vi "OTP - Verify data written.vi"(4 "Read Return":string[](array[string]), 6 "Write Return":string[](array[string]), 9 "Read in":T1[](array[typedef]), 11 "write in":T1[](array[typedef])) -> (0 "# of regs still to be written":i32, 1 "Read out":T1[](array[typedef]), 3 "write out":T1[](array[typedef]))   [LabVIEW 2020]
uses:
  Devices/Controls/Register to Write.ctl
  Devices/PIC-device/PIC-Device.lvclass
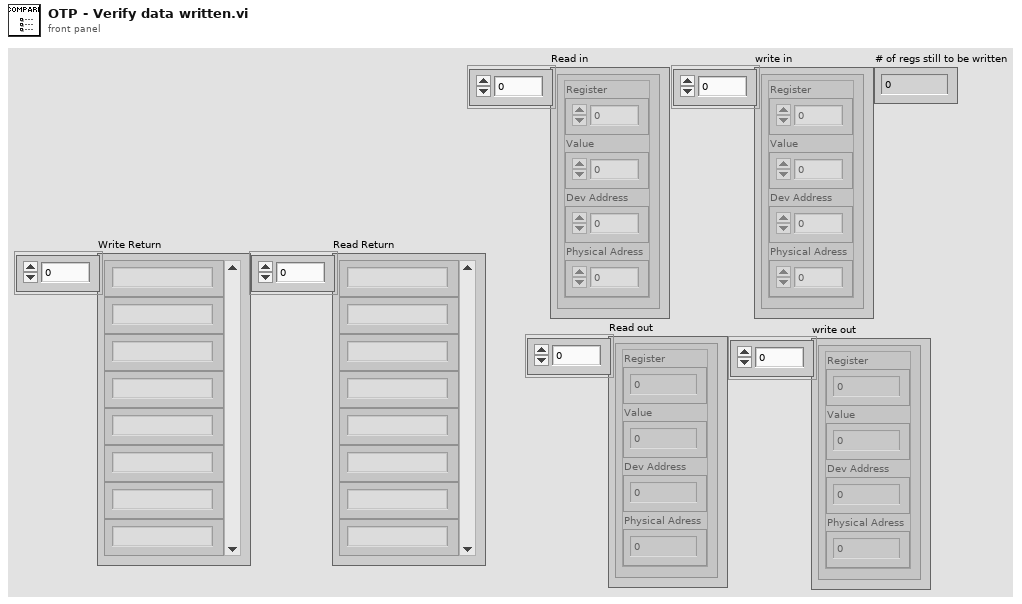
[diagram p1: front panel]
types:
  T1 = typedef "PIC-Device.lvclass/Register to Write.ctl" = cluster{"Register":u32, "Value":u32, "Dev Address":u32, "Physical Adress":u32}
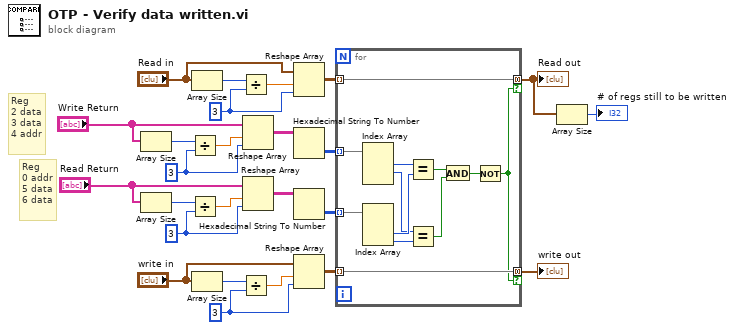
[diagram p0: block diagram]
diagram:
  w4 = 3 ("y")
  w3 = 3 ("y")
  w5 = 3 ("y")
  w6 = 3 ("y")
  # "Reg\n0 addr\n5 data\n6 data"
  # "Reg\n2 data\n3 data\n4 addr"
  n1 = Array Size(array="Write Return") -> (size(s)=w25:i32)
  n2 = Array Size(array="Read Return") -> (size(s)=w21:i32)
  n3 = Divide(x=w25, y=w6) -> (x/y=w24:dbl)
  n4 = Divide(x=w21, y=w5) -> (x/y=w22:dbl)
  n5 = Array Size(array="Read in") -> (size(s)=w18:i32)
  n6 = Array Size(array="write in") -> (size(s)=w17:i32)
  n7 = Divide(x=w18, y=w3) -> (x/y=w19:dbl)
  n8 = Divide(x=w17, y=w4) -> (x/y=w16:dbl)
  n9 = Reshape Array("Write Return", w24, w6) -> (w10:string[][])
  n10 = Reshape Array("Read Return", w22, w5) -> (w8:string[][])
  n11 = Reshape Array("Read in", w19, w3) -> (w13:T1[][])
  n12 = Hexadecimal String To Number(string=w10) -> (number=w9:u32[][])  [unwired: 2 in, 1 out]
  n13 = Hexadecimal String To Number(string=w8) -> (number=w7:u32[][])  [unwired: 2 in, 1 out]
  n14 = Reshape Array("write in", w16, w4) -> (w12:T1[][])
  n15 = for {
    tunnel: w9 -> [w36] mode=indexing
    tunnel: w7 -> [w37] mode=indexing
    tunnel: w13 -> [w30] mode=indexing
    tunnel: w12 -> [w31] mode=indexing
    tunnel: [w31] -> w11 mode=concatenating if=w26
    tunnel: [w30] -> w2 mode=concatenating if=w26
    n16 = Index Array(array=w36) -> (element #1=w28:u32, element #2=w27:u32)  [unwired: 3 in, 1 out]
    n17 = Index Array(array=w37) -> (element #2=w35:u32, element #3=w34:u32)  [unwired: 3 in, 1 out]
    n18 = Equal?(x=w28, y=w35) -> (x = y?=w32:bool)
    n19 = Equal?(x=w27, y=w34) -> (x = y?=w33:bool)
    n20 = And(x=w32, y=w33) -> (x .and. y?=w29:bool)
    n21 = Not(x=w29) -> (.not. x?=w26:bool)
  }
  "Read out" <- w2
  "write out" <- w11
  n22 = Array Size(array=w2) -> (size(s)=→"# of regs still to be written":i32)
